vi "read typedef clusters for channel info.vi"() -> (0 "error out":errorcluster, 2 "> Categorized name list >":string[][](array[string]), 3 "> Uncategorized name list >":string[](array[string]))   [LabVIEW 2013, in "fixed channel tag bus module configuration.lvclass"]
uses:
  fixed channel tag bus module configuration.lvclass
  <vilib>/NI/Tag Bus Module Framework/channel/channel classification.ctl
  <vilib>/NI/Tag Bus Module Framework/channel/TBM channel.lvclass
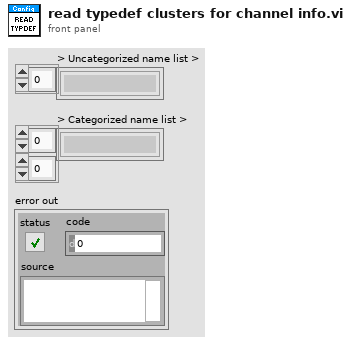
[diagram p1: front panel]
types:
  T1 = typedef "TBM channel.lvclass/channel classification.ctl" = enum16{"input data", "output data", "processing parameter", "processing result"}
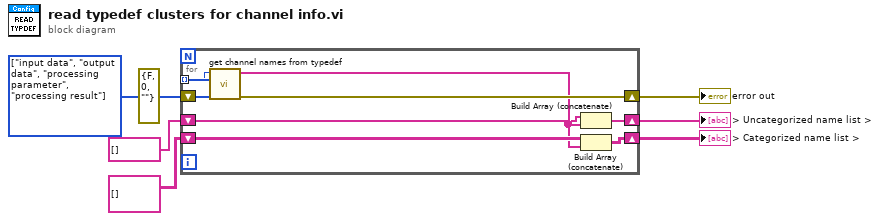
[diagram p0: block diagram]
diagram:
  w4 = T1[] [enum."input data", enum."output data", enum."processing parameter", enum."processing result"] items=["input data", "output data", "processing parameter", "processing result"]
  n1 = for {
    tunnel: w4 -> [w15] mode=indexing
    shift-right: [w14] -> w3
    shift-left: string[][] [] -> [w13]
    shift-right: [w12] -> w7
    shift-left: errorcluster {"status"=FALSE, "code"=0, "source"=""} ("error out") -> [w11]
    shift-right: [w9] -> w6
    shift-left: string[] [] -> [w8]
    n2 = call "get channel names from typedef.vi"("error in (no error)"=w11, "channel classification"=w15) -> ("error out"=w12:errorcluster, "Channel Names"=w10:string[])  [unwired: 8 in]
    n3 = Build Array (concatenate)(w8, w10) -> (w9:string[])
    n4 = Build Array (concatenate)(w13, w10) -> (w14:string[][])
  }
  "error out" <- w7
  "> Uncategorized name list >" <- w6
  "> Categorized name list >" <- w3
